vi "magTerm.vi"() -> ()   [LabVIEW 2012]
uses:
  <userlib>/libdriver_powersupply/libdriver_powersupply.lvlib
panel:
  in  "stop":bool
  out "Array":T1(array[cluster])
  in  "MDS":string="mdsserver:5000"
  in  "Element List":string[](array[string])
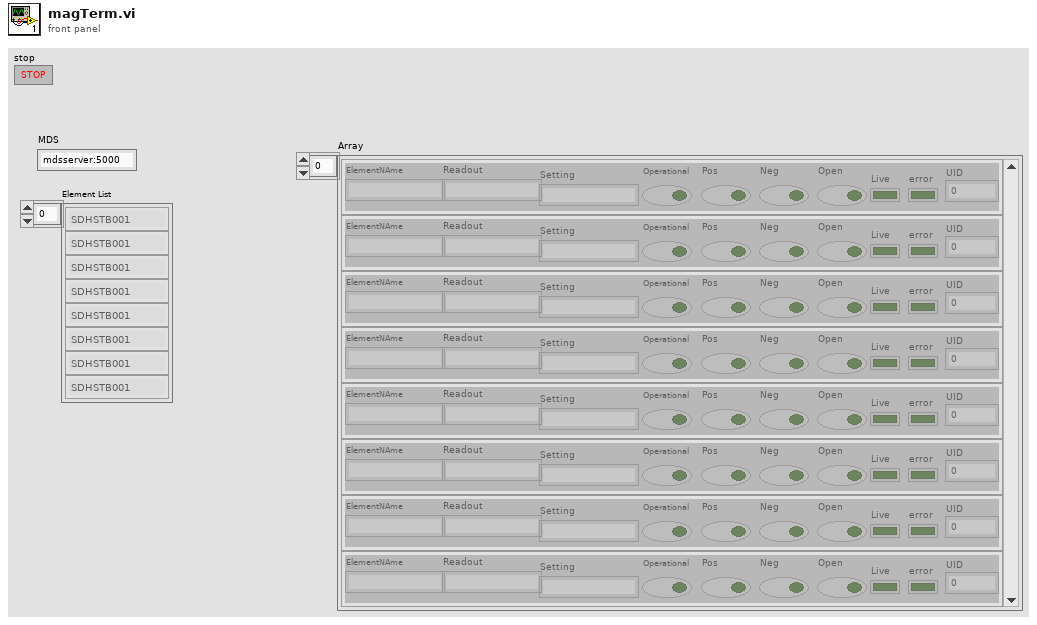
[diagram p1: front panel]
types:
  T1 = cluster{"ElementNAme":string, "Readout":string, "Setting":string, "Operational":bool, "Pos":bool, "Neg ":bool, "Open":bool, "Live":bool, "error":bool, "UID":u32}[]
  T2 = cluster{"ElementNAme":string, "Readout":string, "Setting":string, "Operational":bool, "Pos":bool, "Neg ":bool, "Open":bool, "Live":bool, "error":bool, "UID":u32}
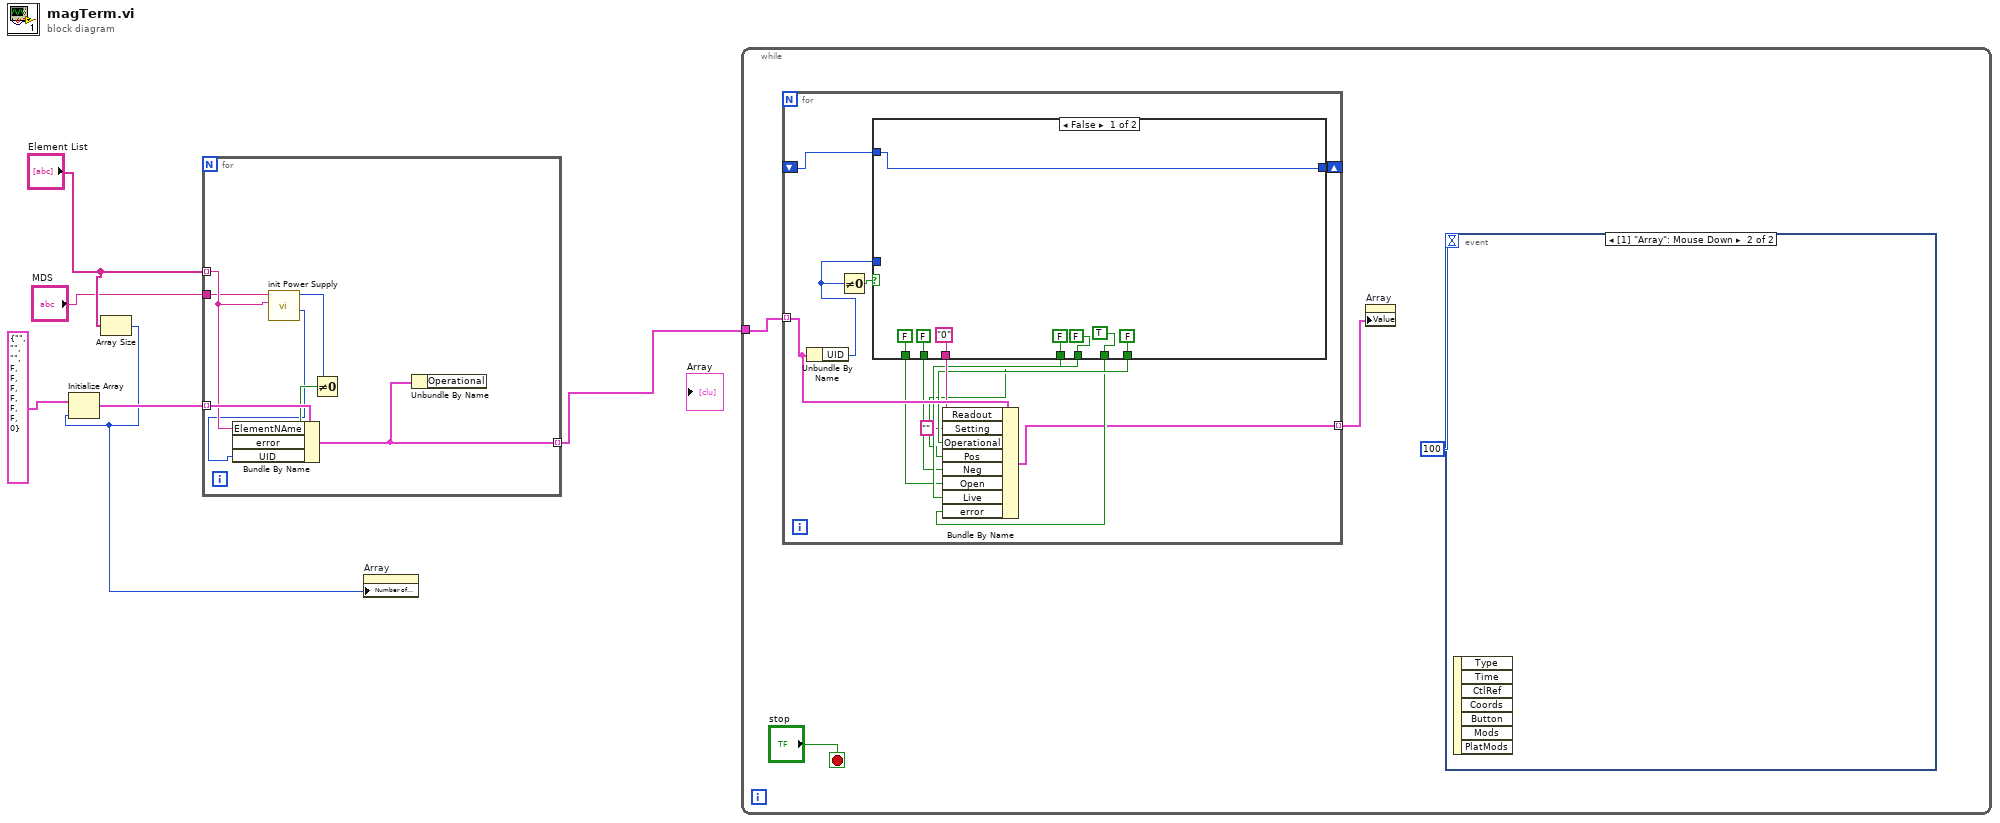
[diagram p0: block diagram]
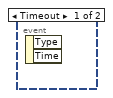
[diagram p2: hidden frame]
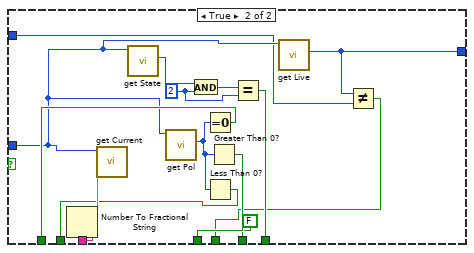
[diagram p3: hidden frame]
diagram:
  n1 = Array Size(array="Element List") -> (size(s)=w1:i32)
  n2 = Initialize Array(T2 {"ElementNAme"="", "Readout"="", "Setting"="", "Operational"=FALSE, "Pos"=FALSE, "Neg "=FALSE, "Open"=FALSE, "Live"=FALSE, "error"=FALSE, "UID"=0} ("magElem"), w1) -> (w4:T1)
  n3 = for {
    tunnel: "Element List" -> [w12] mode=indexing
    tunnel: w4 -> [w13] mode=indexing
    tunnel: "MDS" -> [w11]
    tunnel: [w7] -> w2 mode=indexing
    n4 = call <userlib>:"init Power Supply.vi"("name"=w12, "mds"=w11) -> ("devID out"=w8:u32, "function return"=w10:i32)  [unwired: 8 in]
    n5 = Not Equal To 0?(x=w10) -> (x != 0?=w9:bool)
    n6 = Bundle By Name(cluster=w13, "ElementNAme"=w12, "error"=w9, "UID"=w8) -> (w7:T2)
    n7 = Unbundle By Name(w7) -> ()  [unwired: 1 out]
  }
  n8 = property on="Array" class="Arr (strict)"("Number of Rows"=w1) -> ()  [unwired: 2 in, 2 out]
  n9 = while {
    tunnel: w2 -> [w17]
    stop <- "stop" stop-if-true
    n10 = for {
      tunnel: w17 -> [w29] mode=indexing
      shift-right: [w18] -> _
      shift-left: _ -> [w21]
      tunnel: [w20] -> w15 mode=indexing
      n11 = Unbundle By Name(w29) -> ("UID"=w31:u32)
      n12 = Not Equal To 0?(x=w31) -> (x != 0?=w30:bool)
      n13 = case shown="False" w30 {
        tunnel: w31 -> [_ w43]
        tunnel: ["0" w53] -> w28
        tunnel: [FALSE w49] -> w27
        tunnel: [TRUE FALSE] -> w26
        tunnel: [FALSE w40] -> w25
        tunnel: [FALSE w45] -> w24
        tunnel: [FALSE w48] -> w23
        tunnel: [FALSE w46] -> w22
        tunnel: w21 -> [w32 w41]
        tunnel: [w32 w42] -> w18
        frame False {
        }
        frame True {
          w50 = 2 ("y")
          n14 = call <userlib>:"get Current.vi"("devID"=w43) -> ("current out"=w54:dbl)  [unwired: 9 in, 1 out]
          n15 = Number To Fractional String(number=w54) -> (F-format string=w53:string)  [unwired: 3 in]
          n16 = call <userlib>:"get State.vi"("devID"=w43) -> ("state out"=w52:i32)  [unwired: 9 in, 1 out]
          n17 = call <userlib>:"get Pol.vi"("devID"=w43) -> ("pol out"=w47:i32)  [unwired: 9 in, 1 out]
          n18 = And(x=w52, y=w50) -> (x .and. y?=w51:i32)
          n19 = Equal To 0?(x=w47) -> (x = 0?=w46:bool)
          n20 = Less Than 0?(x=w47) -> (x < 0?=w48:bool)
          n21 = Greater Than 0?(x=w47) -> (x > 0?=w45:bool)
          n22 = Equal?(x=w51, y=w50) -> (x = y?=w49:bool)
          n23 = call <userlib>:"get Live.vi"("devID"=w43) -> ("live out"=w42:i64)  [unwired: 9 in, 1 out]
          n24 = Not Equal?(x=w42, y=w41) -> (x != y?=w40:bool)
        }
      }
      n25 = Bundle By Name(cluster=w29, "Readout"=w28, "Setting"="", "Operational"=w27, "Pos"=w24, "Neg"=w23, "Open"=w22, "Live"=w25, "error"=w26) -> (w20:T2)
    }
    n26 = property on="Array" class="Arr (strict)"("Value"=w15) -> ()  [unwired: 2 in, 2 out]
    n27 = event shown="[1] \"Array\": Mouse Down" {
      selector: _ -> [_ _]
      dyn-events: _ -> [_ _]
      timeout: 100 -> [_ _]
      event Timeout {
        n28 = event-data() -> ()  [unwired: 1 in, 2 out]
      }
      event "Array": Mouse Down {
        n29 = event-data() -> ()  [unwired: 1 in, 7 out]
      }
    }
  }
